vi "Set State Queue.vi"(0 "reference in":refnum<class "Generic Utilities.lvclass">, 5 "error in (no error)":errorcluster, 7 "State Queue Options":enum16{"Replace", "Append", "Prepend"}(ring), 9 "State Queue":string[](array[string])) -> (14 "reference out":refnum<class "Generic Utilities.lvclass">, 19 "error out":errorcluster)   [LabVIEW 2020, in "Generic Utilities.lvclass"]
doc: "This will replace, prepend or append an array of states to the state queue."
uses:
  Generic Utilities.lvclass
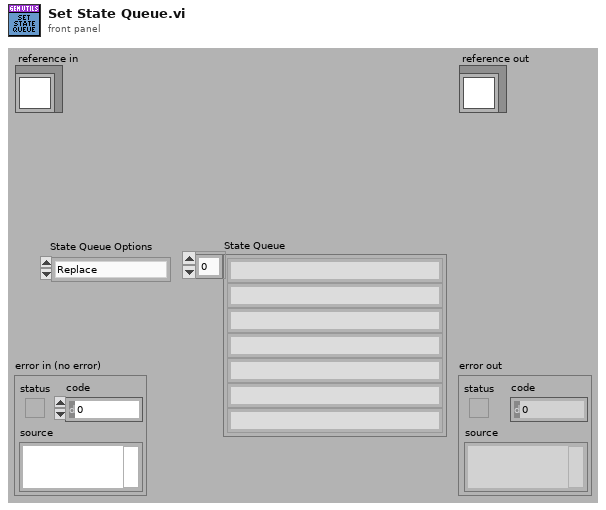
[diagram p1: front panel]
types:
  T1 = typedef "Generic Utilities.lvclass/ObjectAttributesRef.ctl" = refnum<data-value>
  T2 = typedef "Generic Utilities.lvclass/ObjectAttributes.ctl" = cluster{"GUI Parameters":T3, "State Machine Control":cluster{"Timeout":i32, "State Queue":string[], "State History":string[], "State History Length":i32}, "Logging File Path":path, "OBJ not a refnum?":bool, "Timer Start":timestamp, "FP Refnums":T4}
  T3 = typedef "Generic Utilities.lvclass/GUI Parameters.ctl" = cluster{"Application Name":string, "GUI VI Ref":refnum<vi>, "Close Panel?":bool, "Message Window ref":refnum<vi>, "Version #":string}
  T4 = typedef "Generic Utilities.lvclass/FP Refnums.ctl" = cluster{"Panel refnum":refnum<vi>, "Control Labels":string[], "Refnums":refnum<vi>[]}
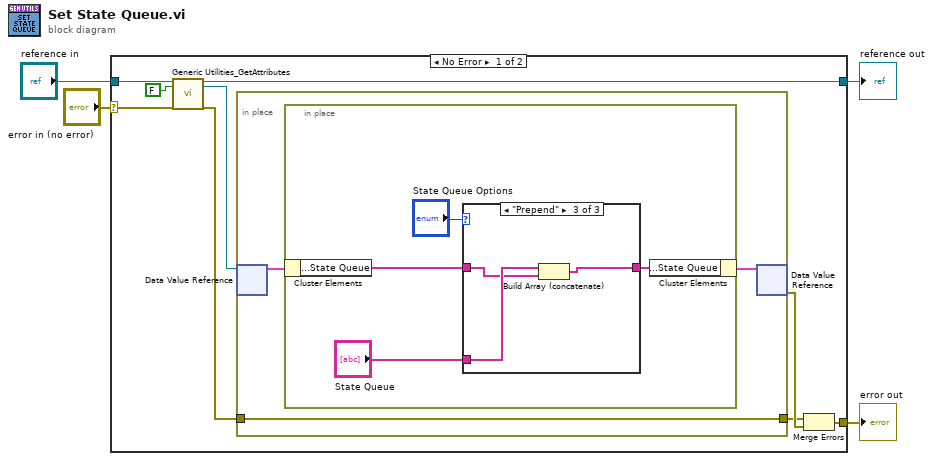
[diagram p0: block diagram]
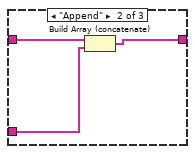
[diagram p3: hidden frame]
diagram:
  n1 = case shown="No Error" "error in (no error)" {
    selector: "error in (no error)" -> [w8 w29]
    tunnel: [w13 w29] -> w3
    tunnel: [w6 w28] -> w1
    tunnel: "reference in" -> [w10 w28]
    frame No Error {
      n2 = call "Generic Utilities_GetAttributes.vi"("reference in"=w10, "return data? (T)"=FALSE, "error in (no error)"=w8) -> ("reference out"=w6:refnum<class "Generic Utilities.lvclass">, "attributes ref"=w5:T1, "error out"=w7:errorcluster)  [unwired: 13 in, 1 out]
      n3 = in-place {
        in-place-border: w7 -> [w14]
        in-place-border: [w14] -> w11
        n4 = in-place-dvr #1(w5) -> (w15:T2)  [unwired: 1 out]
        n5 = in-place {
          n6 = in-place-cluster #2(w15) -> ("State Machine Control.State Queue"=w17:string[])
          n7 = case shown="\"Prepend\"" "State Queue Options" {
            tunnel: [w21 w22 w27] -> w19
            tunnel: "State Queue" -> [w21 w23 w26]
            tunnel: w17 -> [_ w24 w25]
            frame "Replace", Default {
            }
            frame "Append" {
              n8 = Build Array (concatenate)(w24, w23) -> (w22:string[])
            }
            frame "Prepend" {
              n9 = Build Array (concatenate)(w26, w25) -> (w27:string[])
            }
          }
          n10 = in-place-cluster #2("State Machine Control.State Queue"=w19) -> (w16:T2)
        }
        n11 = in-place-dvr #1(w16) -> (w12:errorcluster)  [unwired: 1 out]
      }
      n12 = Merge Errors(w11, w12) -> (w13:errorcluster)
    }
    frame Error {
    }
  }
  "error out" <- w3
  "reference out" <- w1
